vi "config.vi"(8 "error in (no error)":errorcluster, 10 "confData":T1, 11 "Logger in":refnum<class "Logger.lvclass">) -> (0 "error out":errorcluster, 3 "Logger out":refnum<class "Logger.lvclass">)   [LabVIEW 2018, in "Logger.lvclass"]
doc: "Configure the Logger."
uses:
  Logger.lvclass
  Logger.lvclass/Logger.ctl
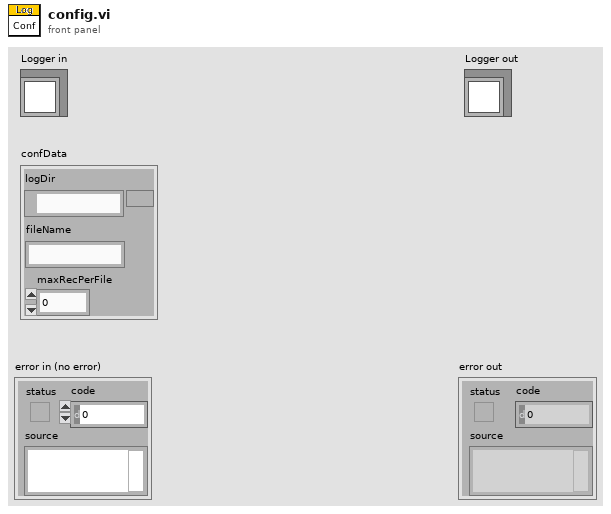
[diagram p1: front panel]
types:
  T1 = cluster{"logDir":path, "fileName":string, "maxRecPerFile":u32}
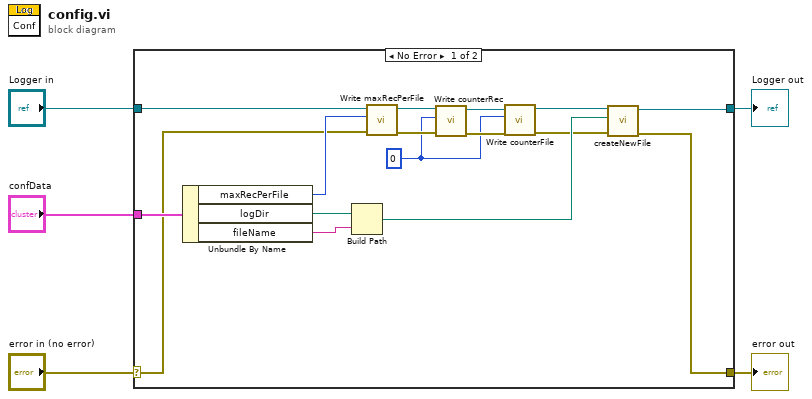
[diagram p0: block diagram]
diagram:
  n1 = case shown="No Error" "error in (no error)" {
    selector: "error in (no error)" -> [w18 w23]
    tunnel: [w12 w23] -> w4
    tunnel: [w11 w22] -> w2
    tunnel: "Logger in" -> [w20 w22]
    tunnel: "confData" -> [w21 _]
    frame No Error {
      w6 = u32 0 ("counterRec")
      n2 = Unbundle By Name(w21) -> ("maxRecPerFile"=w19:u32, "logDir"=w17:path, "fileName"=w16:string)
      n3 = Build Path(base path=w17, name or relative path=w16) -> (appended path=w15:path)
      n4 = call "Write maxRecPerFile.vi"("error in (no error)"=w18, "maxRecPerFile"=w19, "Logger in"=w20) -> ("error out"=w7:errorcluster, "Logger out"=w10:refnum<class "Logger.lvclass">)  [unwired: 7 in]
      n5 = call "Write counterRec.vi"("error in (no error)"=w7, "counterRec"=w6, "Logger in"=w10) -> ("error out"=w8:errorcluster, "Logger out"=w9:refnum<class "Logger.lvclass">)  [unwired: 7 in]
      n6 = call "Write counterFile.vi"("error in (no error)"=w8, "counterFile"=w6, "Logger in"=w9) -> ("error out"=w13:errorcluster, "Logger out"=w14:refnum<class "Logger.lvclass">)  [unwired: 7 in]
      n7 = call "createNewFile.vi"("error in (no error)"=w13, "filePath"=w15, "Logger in"=w14) -> ("error out"=w12:errorcluster, "Logger out"=w11:refnum<class "Logger.lvclass">)  [unwired: 7 in]
    }
    frame Error {
    }
  }
  "error out" <- w4
  "Logger out" <- w2
